vi "Hide Unused.vi"(0 "Display State":T1 caption="State") -> (15 "error out":errorcluster)   [LabVIEW 2020, in "PXISlotGP.xctl"]
uses:
  PXISlotGP.xctl
  State.ctl
  PXISlot XControl/Connector Type.ctl
  AOAIRefs.ctl
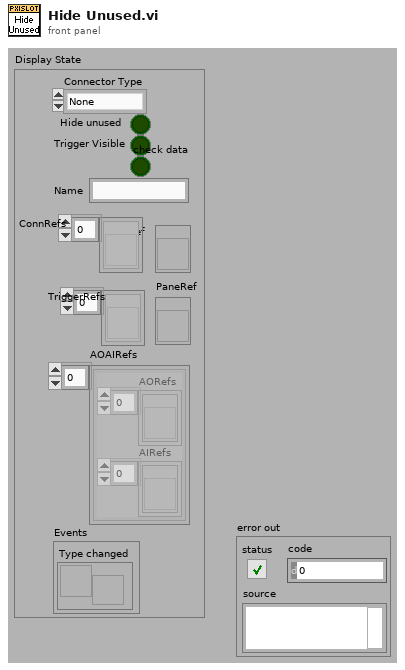
[diagram p1: front panel]
types:
  T1 = typedef "PXISlotGP.xctl/State.ctl" = cluster{"Connector Type":T2, "Hide unused":bool, "Trigger Visible":bool, "TabRef":refnum<vi>, "ConnRefs":refnum<vi>[], "PaneRef":refnum<vi>, "AOAIRefs":T3[], "TriggerRefs":refnum<vi>[], "check data":bool, "Name":string, "Events":cluster{"Type changed":refnum<user-event>}}
  T2 = typedef "Connector Type.ctl" = enum16{"None", "PXI-4461", "BNC-2110", "BNC-2090", "PXIe-4463", "PXIe-4464"}
  T3 = typedef "AOAIRefs.ctl" = cluster{"AORefs":refnum<vi>[], "AIRefs":refnum<vi>[]}
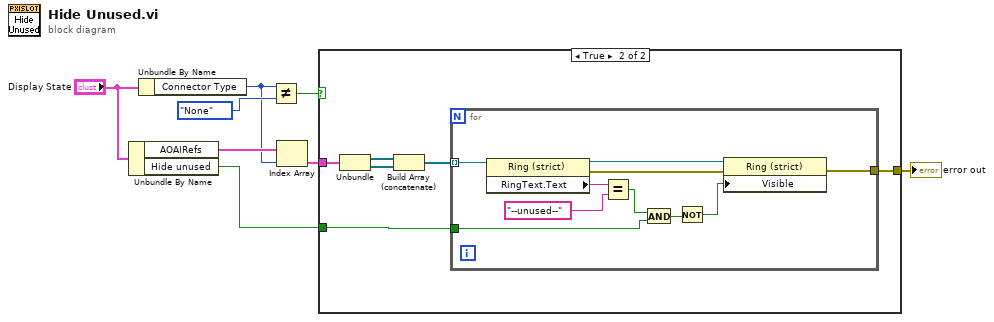
[diagram p0: block diagram]
diagram:
  n1 = Unbundle By Name("Display State") -> ("AOAIRefs"=w5:T3[], "Hide unused"=w4:bool)
  n2 = Unbundle By Name("Display State") -> ("Connector Type"=w2:T2)
  n3 = Not Equal?(x=w2, y=Connector_Type."None") -> (x != y?=w7:bool)
  n4 = Index Array(array=w5, index=w2) -> (element=w6:T3)
  n5 = case shown="True" w7 {
    tunnel: w6 -> [_ w14]
    tunnel: w4 -> [_ w10]
    tunnel: [_ w9] -> w1
    frame False {
    }
    frame True {
      n6 = Unbundle(w14) -> ("AORefs"=w13:refnum<vi>[], "AIRefs"=w12:refnum<vi>[])
      n7 = Build Array (concatenate)(w13, w12) -> (w11:refnum<vi>[])
      n8 = for {
        tunnel: w11 -> [w23] mode=indexing
        tunnel: w10 -> [w24]
        tunnel: [w15] -> w9
        n9 = property class="Ring (strict)"(reference=w23) -> (reference out=w20:refnum<vi>, error out=w18:errorcluster, "RingText.Text"=w22:string)  [unwired: 1 in]
        n10 = Equal?(x=w22, y="--unused--") -> (x = y?=w17:bool)
        n11 = And(x=w17, y=w24) -> (x .and. y?=w19:bool)
        n12 = Not(x=w19) -> (.not. x?=w16:bool)
        n13 = property class="Ring (strict)"(reference=w20, error in=w18, "Visible"=w16) -> (error out=w15:errorcluster)  [unwired: 1 out]
      }
    }
  }
  "error out" <- w1
